vi "Set Temp.vi"(1 "Rate":dbl=10.0, 2 "Temperature":dbl=300.0) -> ()   [LabVIEW 2013]
uses:
  PPMS Global.vi
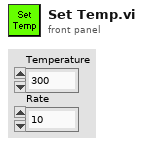
[diagram p1: front panel]
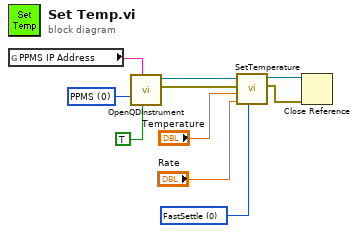
[diagram p0: block diagram]
diagram:
  w1 = 0 items=["FastSettle", "NoOvershoot"] ("Approach")
  w9 = 0 items=["PPMS", "VersaLab", "DynaCool", "SVSM"] ("Instrument\nType")
  n1 = global read "PPMS Global.vi" "PPMS IP Address"() -> (w8:string)
  n2 = call "OpenQDInstrument.vi"("Remote"=TRUE, "IP Address"=w8, "Instrument Type"=w9) -> ("error out"=w6:errorcluster, "Instrument Ref"=w7:refnum<k24>)  [unwired: 5 in]
  n3 = call "SetTemperature.vi"("Approach"=w1, "Rate"="Rate", "Temperature"="Temperature", "error in (no error)"=w6, "Instrument Ref In"=w7) -> ("error out"=w4:errorcluster, "Instrument Ref Out"=w5:refnum<k24>)  [unwired: 2 in, 1 out]
  n4 = Close Reference(reference=w5, error in (no error)=w4) -> ()  [unwired: 1 out]
